vi "LRMS_Scan_Test.vi"() -> ()   [LabVIEW 2019]
uses:
  <instrlib>/niSwitch/niSwitch.llb/niSwitch Connect Channels (Multiple).vi
panel:
  out "IVI Match":string[][](array[string])=[["SwitchBlock1Dev1", "SwitchBlock1Dev1", "2526_1"], ["2526_1", "SwitchBlock1Dev1", "SwitchBlock1Dev1"], ["SwitchBlock1Dev1", "SwitchBlock1Dev1", "2526_1"], ["2526_1", "SwitchBlock1Dev1", "SwitchBlock1Dev1"], ["SwitchBlock1Dev1", "SwitchBlock1Dev1", "2526_1"], ["SwitchBlock1Dev1", "SwitchBlock1Dev1", "2526_1"], ["SwitchBlock1Dev1", "SwitchBlock1Dev1", "2526_1"]]
  out "Array":refnum<k15>[](array[refnum])=["SwitchBlock1Dev1", "SwitchBlock1Dev1", "2526_1"]
  in  "Channel Index":i32=6
  out "Current Connection":string[](array[string])=["[ab0->card1r0->c30]", "[ab1->card1r1->c31]", "[com->ch76]"]
  out "Channel Specs":string[][](array[string])=[["[ab0->card1r0->c2]", "[ab1->card1r1->c3]", "[com->ch70]"], ["[com->ch71]", "[ab0->card1r0->c6]", "[ab1->card1r1->c7]"], ["[ab0->card1r0->c10]", "[ab1->card1r1->c11]", "[com->ch72]"], ["[com->ch73]", "[ab0->card1r0->c14]", "[ab1->card1r1->c15]"], ["[ab0->card1r0->c18]", "[ab1->card1r1->c19]", "[com->ch74]"], ["[ab0->card1r0->c22]", "[ab1->card1r1->c23]", "[com->ch75]"], ["[ab0->card1r0->c30]", "[ab1->card1r1->c31]", "[com->ch76]"]]
  in  "Channel List":string[](array[string])=["Ch0", "ch1", "ch2", "ch3", "ch4", "ch5", "ch6"]
  in  "file path (dialog if empty)":path=path "/home/lvuser/Chad_Test.csv"
  in  "MUX Devices":refnum<k15>[](array[refnum])=["SwitchBlock1Dev1", "2526_1"]
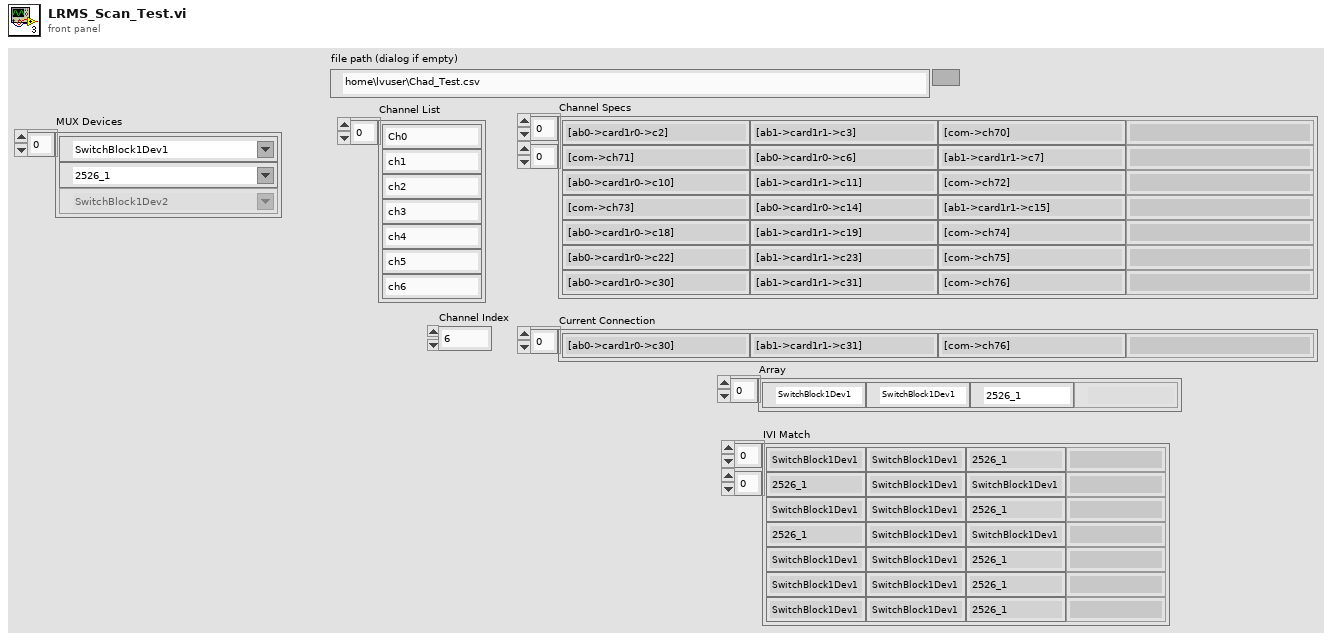
[diagram p1: front panel]
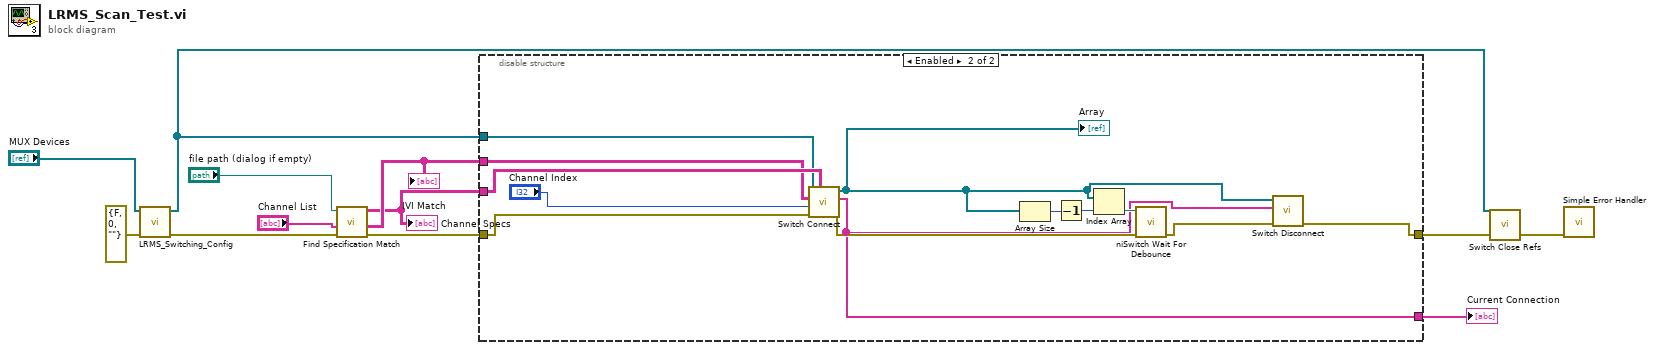
[diagram p0: block diagram]
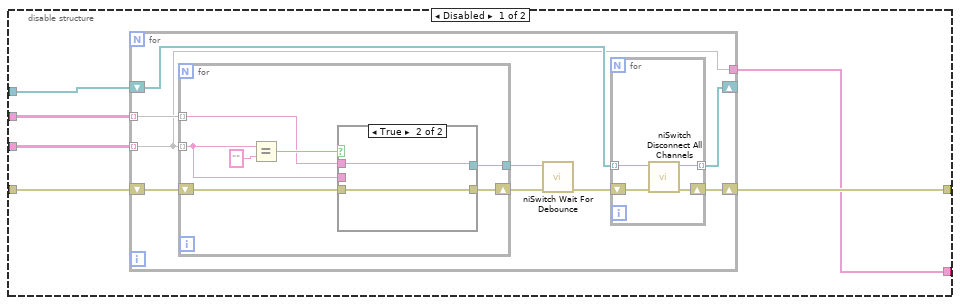
[diagram p2: hidden frame]
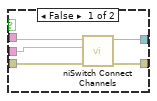
[diagram p3: hidden frame]
diagram:
  n1 = call "LRMS_Switching_Config.vi"("error in (no error)"=errorcluster {"status"=FALSE, "code"=0, "source"=""} ("error out"), "Sense MUX Devices"="MUX Devices") -> ("error out"=w9:errorcluster, "Array"=w1:refnum<k15>[])  [unwired: 8 in]
  n2 = call "Find Specification Match.vi"("error in (no error)"=w9, "Channel List"="Channel List", "file path (dialog if empty)"="file path (dialog if empty)") -> ("error out"=w7:errorcluster, "IVI Specifications"=w5:string[][], "Channel Specs"=w4:string[][])  [unwired: 5 in]
  "Channel Specs" <- w4
  "IVI Match" <- w5
  n3 = disable-structure shown="Enabled" {
    disable-tunnel: w7 -> [w18 w53]
    disable-tunnel: [w17 w52] -> w3
    disable-tunnel: w4 -> [w16 w56]
    disable-tunnel: w5 -> [w15 w55]
    disable-tunnel: w1 -> [w14 w54]
    disable-tunnel: [w13 w46] -> w2
    frame Disabled {
      n4 = for {
        tunnel: w15 -> [w24] mode=indexing
        tunnel: w16 -> [w19] mode=indexing
        shift-right: [w21] -> _
        shift-left: w14 -> [w22]
        shift-right: [w20] -> w17
        shift-left: w18 -> [w27]
        tunnel: [w19] -> w13
        n5 = for {
          tunnel: w24 -> [w32] mode=indexing
          tunnel: w19 -> [w33] mode=indexing
          tunnel: [w37] -> w26
          shift-right: [w36] -> w25
          shift-left: w27 -> [w38]
          n6 = Equal?(x=w33, y="") -> (x = y?=w34:bool)
          n7 = case shown="True" w34 {
            tunnel: w38 -> [w43 w45]
            tunnel: [w42 w44] -> w37
            tunnel: [w41 w45] -> w36
            tunnel: w33 -> [w40 _]
            tunnel: w32 -> [w39 w44]
            frame False {
              n8 = call-poly <instrlib>:"niSwitch Connect Channels.vi"("error in (no error)"=w43, "connection list"=w40, "instrument handle"=w39) -> ("error out"=w41:errorcluster, "instrument handle out"=w42:refnum<k15>)  [unwired: 7 in]
            }
            frame True {
            }
          }
        }
        n9 = call <instrlib>:"niSwitch Wait For Debounce.vi"("error in (no error)"=w25, "instrument handle"=w26) -> ("error out"=w23:errorcluster)  [unwired: 8 in, 1 out]
        n10 = for {
          tunnel: w22 -> [w30] mode=indexing
          shift-right: [w29] -> w20
          shift-left: w23 -> [w31]
          tunnel: [w28] -> w21 mode=indexing
          n11 = call <instrlib>:"niSwitch Disconnect All Channels.vi"("error in (no error)"=w31, "instrument handle"=w30) -> ("error out"=w29:errorcluster, "instrument handle out"=w28:refnum<k15>)  [unwired: 8 in]
        }
      }
    }
    frame Enabled {
      n12 = call "Switch Connect.vi"("Channel Specs"=w56, "error in (no error)"=w53, "Channel Index"="Channel Index", "IVI Specifications"=w55, "Switch Refs"=w54) -> ("error out"=w51:errorcluster, "Channels Connected"=w46:string[], "Refs Connected"=w48:refnum<k15>[])  [unwired: 4 in]
      "Array" <- w48
      n13 = Array Size(array=w48) -> (size(s)=w58:i32)
      n14 = Decrement(x=w58) -> (x-1=w49:i32)
      n15 = Index Array(array=w48, index=w49) -> (element=w47:refnum<k15>)
      n16 = call <instrlib>:"niSwitch Wait For Debounce.vi"("error in (no error)"=w51, "instrument handle"=w47) -> ("error out"=w50:errorcluster)  [unwired: 8 in, 1 out]
      n17 = call "Switch Disconnect.vi"("error in (no error)"=w50, "Channels Connected"=w46, "Switch Refs"=w48) -> ("error out"=w52:errorcluster)  [unwired: 8 in]
    }
  }
  "Current Connection" <- w2
  n18 = call "Switch Close Refs.vi"("error in (no error)"=w3, "Switch Refs"=w1) -> ("error out"=w6:errorcluster)  [unwired: 9 in]
  n19 = call <vilib>:"Simple Error Handler.vi"("error in (no error)"=w6) -> ()  [unwired: 4 in, 5 out]
